vi "PromptForPlugin.vi"(0 "Enable":bool=TRUE, 1 "Measurement Plug-in":string, 5 "error in (no error)":errorcluster) -> (17 "Measurement Plug-in":string, 18 "OK":bool, 19 "error out":errorcluster)   [LabVIEW 2020]
doc: "Displays a standard dialog box that prompts users to enter information, such as a user name and password.\n--------------------\n\nThis Express VI is configured as follows:\n\nMessage to Display to the User:Enter the Measurement Plug-in to create\nThe inputs are: \nText Entry Box: Measurement Plug-in"
panel:
  out "String":string="Enter the Measurement Plug-in to create"
  in  "Cancel":bool
  in  "OK2":bool
  in  "OK1":bool
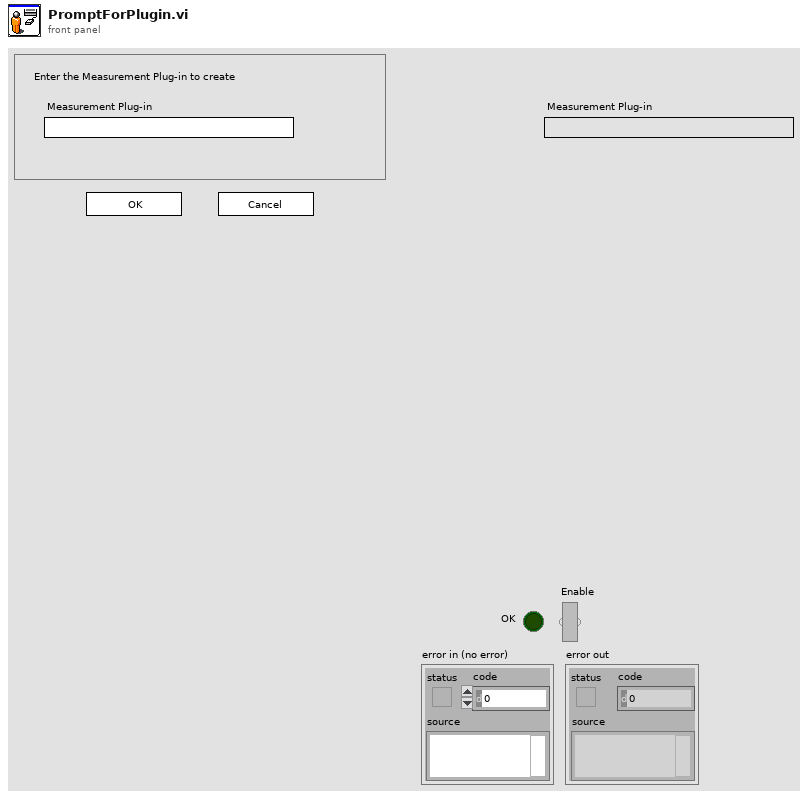
[diagram p1: front panel]
types:
  T1 = cluster{"Input Name":string, "Input Data Type":i32}[]
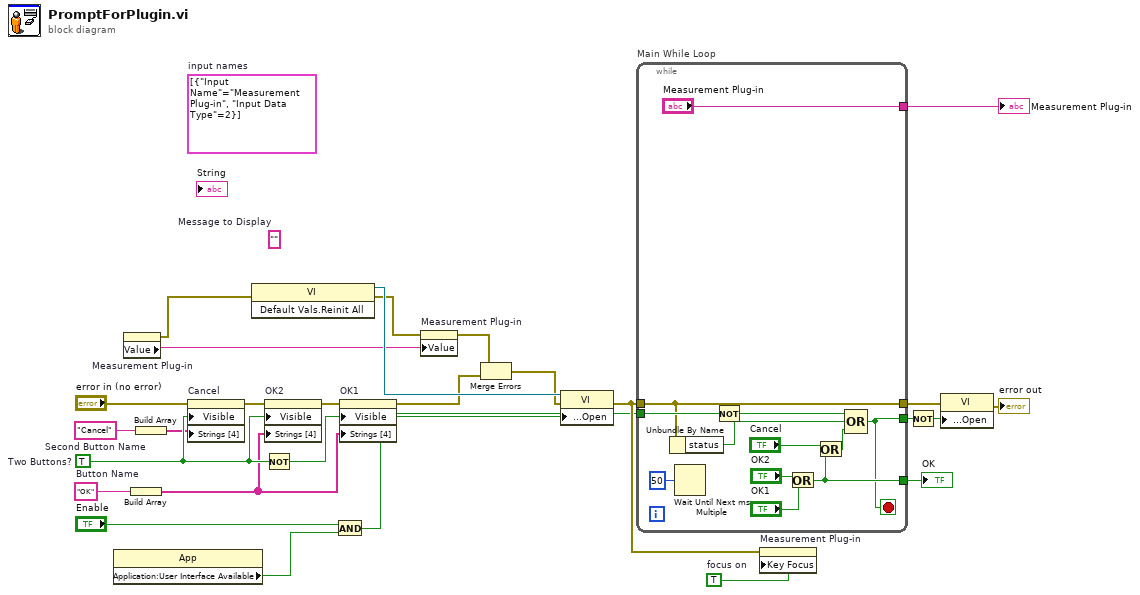
[diagram p0: block diagram]
diagram:
  w7 = TRUE  # focus on
  (unwired) T1 [{"Input Name"="Measurement Plug-in", "Input Data Type"=2}]  # input names
  w19 = "Cancel"  # Second Button Name
  w17 = "OK"  # Button Name
  (unwired) ""  # Message to Display
  w27 = TRUE  # Two Buttons?
  n1 = property class="App"() -> ("Application:User Interface Available"=w10:bool)  [unwired: 2 in, 2 out]
  n2 = property on="Measurement Plug-in" class="Str"() -> (error out=w6:errorcluster, "Value"=w4:string)  [unwired: 2 in, 1 out]
  n3 = Build Array(w17) -> (w18:string[])
  n4 = Build Array(w19) -> (w20:string[])
  n5 = property on="Cancel" class="Bool"(error in="error in (no error)", "Visible"=w27, "Strings [4]"=w20) -> (error out=w24:errorcluster)  [unwired: 1 in, 1 out]
  n6 = invoke class="VI" method="Default Vals.Reinit All"(error in=w6) -> (reference out=w9:refnum<vi>, error out=w5:errorcluster)  [unwired: 2 in, 1 out]
  n7 = Not(x=w27) -> (.not. x?=w25:bool)
  n8 = property on="OK2" class="Bool"(error in=w24, "Visible"=w27, "Strings [4]"=w18) -> (error out=w23:errorcluster)  [unwired: 1 in, 1 out]
  n9 = And(x="Enable", y=w10) -> (x .and. y?=w11:bool)
  n10 = property on="OK1" class="Bool"(error in=w23, "Visible"=w25, "Strings [4]"=w18) -> (error out=w2:errorcluster)  [unwired: 1 in, 1 out]
  n11 = property on="Measurement Plug-in" class="Str"(error in=w5, "Value"=w4) -> (error out=w3:errorcluster)  [unwired: 1 in, 1 out]
  n12 = Merge Errors(w3, w2) -> (w1:errorcluster)
  n13 = property class="VI"(reference=w9, error in=w1, "Front Panel Window:Open"=w11) -> (error out=w16:errorcluster)  [unwired: 1 out]
  n14 = while "Main While Loop" {
    tunnel: [w36] -> w26
    tunnel: w11 -> [w34]
    tunnel: [w32] -> w21
    tunnel: w16 -> [w31]
    tunnel: [w31] -> w14
    tunnel: ["Measurement Plug-in"] -> w8
    stop <- w32 stop-if-true
    n15 = Unbundle By Name(w31) -> ("status"=w29:bool)
    n16 = Wait Until Next ms Multiple(millisecond multiple=u32 50) -> ()  [unwired: 1 out]
    n17 = Not(x=w34) -> (.not. x?=w33:bool)
    n18 = Or(x="OK2", y="OK1") -> (x .or. y?=w36:bool)
    n19 = Or(x="Cancel", y=w36) -> (x .or. y?=w30:bool)
    n20 = Compound Arithmetic op=OR(w33, w29, w30) -> (w32:bool)
  }
  "OK" <- w26
  "Measurement Plug-in" <- w8
  n21 = property on="Measurement Plug-in" class="Str"(error in=w16, "Key Focus"=w7) -> ()  [unwired: 1 in, 2 out]
  n22 = Not(x=w21) -> (.not. x?=w22:bool)
  n23 = property class="VI"(error in=w14, "Front Panel Window:Open"=w22) -> (error out=→"error out":errorcluster)  [unwired: 1 in, 1 out]
